vi "CallerToArray.vi"(11 "String":string) -> (3 "Called":string)   [LabVIEW 2018, in "TracerLibrary.lvlib" / "Tracer.lvclass"]
uses:
  Tracer.lvclass
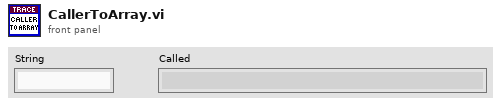
[diagram p1: front panel]
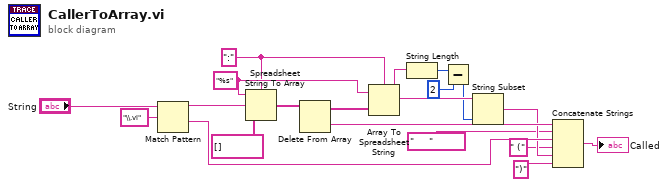
[diagram p0: block diagram]
diagram:
  w13 = "%s" ("format string")
  w12 = ":" ("delimiter (Tab)")
  n1 = Match Pattern(string="String", regular expression="\\.vi") -> (before substring=w15:string, after substring=w9:string)  [unwired: 1 in, 2 out]
  n2 = Spreadsheet String To Array(delimiter (Tab)=w12, format string=w13, spreadsheet string=w15, array type (2D Dbl)=string[] []) -> (array=w16:string[])
  n3 = Delete From Array(array=w16) -> (deleted portion=w10:string, array with subset deleted=w14:string[])  [unwired: 2 in]
  n4 = Array To Spreadsheet String(delimiter (Tab)=w12, array=w14, 3:w13) -> (spreadsheet string=w11:string)
  n5 = String Length(string=w11) -> (length=w6:i32)
  n6 = Subtract(x=w6, y=2) -> (x-y=w4:i32)
  n7 = String Subset(string=w11, length (rest)=w4) -> (substring=w8:string)  [unwired: 1 in]
  n8 = Concatenate Strings(w10, "     " ("string"), w9, " (" ("string"), w8, ")" ("string")) -> (→"Called":string)
